vi "vms_monitorCommand_stop.vi"(8 "error in (no error)":errorcluster, 11 "command_stop_Ctl":T1) -> (0 "error out":errorcluster, 2 "function return":i32, 3 "command_stop_Ctl out":T1)   [LabVIEW 2016, in "SALLV_vms.lvlib"]
doc: "int vms_shm_monitorCommand_stopLV(vms_command_stopLV *command_stop_Ctl );"
uses:
  SALLV_vms.lvlib
  DataTypes/command_stop.ctl
  SALLV_vms.so
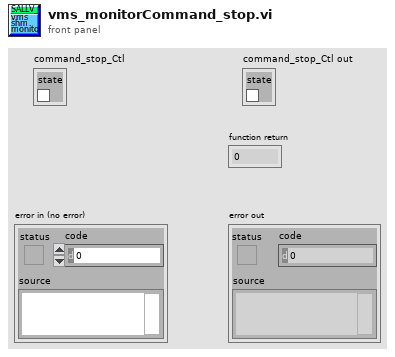
[diagram p1: front panel]
types:
  T1 = typedef "SALLV_vms.lvlib/command_stop.ctl" = cluster{"state":bool}
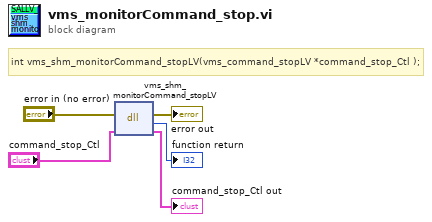
[diagram p0: block diagram]
diagram:
  # "int vms_shm_monitorCommand_stopLV(vms_command_stopLV *command_stop_Ctl );"
  n1 = dll-call lib="opt/CODE/SALLV_vms/SALLV_vms.*" fn="vms_shm_monitorCommand_stopLV"(error in="error in (no error)", "command_stop_Ctl"="command_stop_Ctl") -> (error out=→"error out":errorcluster, →"function return":i32, "command_stop_Ctl"=→"command_stop_Ctl out":T1)  [unwired: 2 in, 1 out]
